vi "MyGlobal2.vi"() -> ()   [LabVIEW 2017]
uses:
  MyGlobal-Global.vi
panel:
  out "布尔":bool
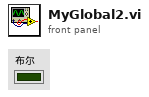
[diagram p1: front panel]
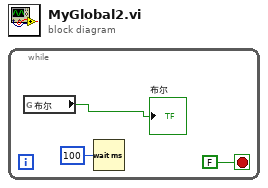
[diagram p0: block diagram]
diagram:
  n1 = while {
    stop <- FALSE stop-if-true
    n2 = global read "MyGlobal-Global.vi" "布尔"() -> (→"布尔":bool)
    n3 = Wait (ms)(milliseconds to wait=u32 100 ("等待时间（毫秒）")) -> ()  [unwired: 1 out]
  }
